vi "Enum Cases.vi"   [LabVIEW 2023]
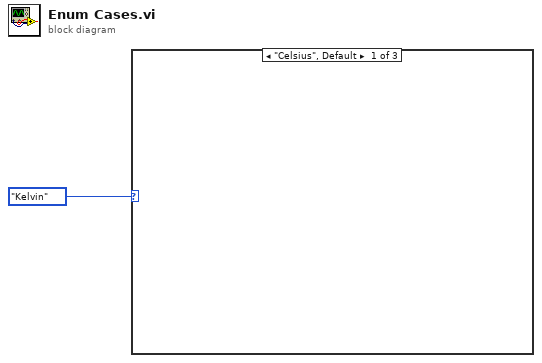
[diagram p0: block diagram]
diagram:
  n1 = case shown="\"Celsius\", Default" enum16{"Celsius", "Fahrenheit", "Kelvin"}."Kelvin" {
    frame "Celsius", Default {
    }
    frame "Fahrenheit" {
    }
    frame "Kelvin" {
    }
  }
